vi "SV TDMS Write Waveform (SGL) (N Ch).vi"(0 "tdms file":refnum<k34>, 1 "write channel properties":bool=TRUE, 5 "group name in":string="Waveforms", 7 "channel names in":string[](array[string]), 9 "scaled signals":waveform(sgl)[](array[waveform]), 11 "error in":errorcluster) -> (4 "tdms file out":refnum<k34>, 6 "group name out":string, 8 "channel names out":string[](array[string]), 15 "error out":errorcluster)   [LabVIEW 2017]
doc: "Writes data to the specified .tdms file in a format specific to the polymorphic instance. Wire data to the <B>scaled signal [EU]</B> input to determine the polymorphic instance to use or manually select the instance."
uses:
  <vilib>/addons/_NISVFA/_Shared subVIs/Controls/LV Datatypes.ctl
  <vilib>/addons/_NISVFA/_Shared subVIs/Controls/NI Function Type.ctl
  <vilib>/addons/_NISVFA/_Shared subVIs/Controls/NI Function SubType.ctl
  <vilib>/addons/_NISVFA/_Shared subVIs/Controls/svc_X-Axis Units.ctl
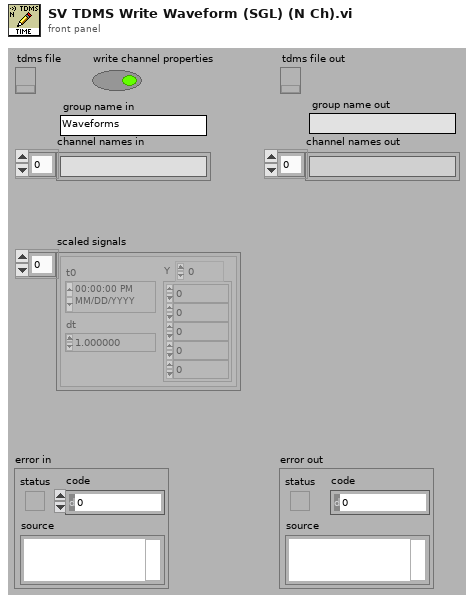
[diagram p1: front panel]
types:
  T1 = typedef "NI Function Type.ctl" = u16
  T2 = typedef "NI Function SubType.ctl" = u16
  T3 = typedef "svc_X-Axis Units.ctl" = u16
  T4 = cluster{"function type":T1, "function subtype":T2, "X-dimension":T3}
  T5 = cluster{"X-axis label":string, "X-unit string":string, "Y-axis label":string, "Y-unit string":string}
  T6 = typedef "LV Datatypes.ctl" = i32
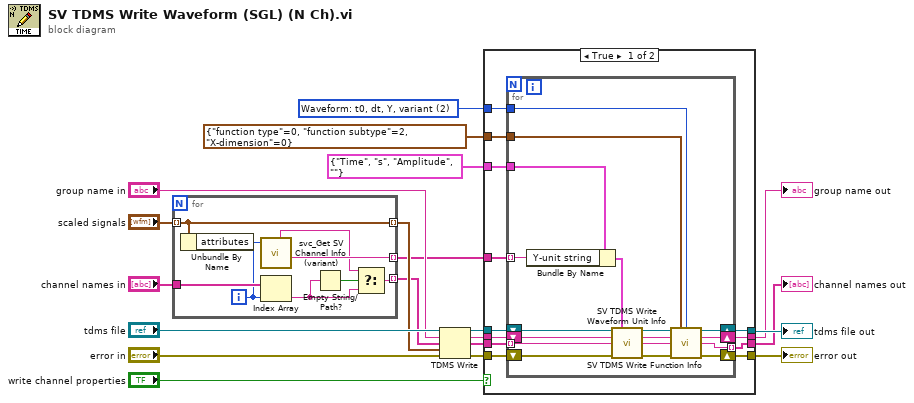
[diagram p0: block diagram]
diagram:
  w1 = T6 2 items=["String: abc"=-2, "Boolean: True or False"=-1, "Scalar: y"=0, "Array: Y"=1, "Waveform: t0, dt, Y, variant"=2, "Cluster: x0, dx, Y"=3, "Cluster: X, Y"=4, "Waterfall"=5, "Colormap"=6] ("LabVIEW datatype")
  n1 = for {
    tunnel: "scaled signals" -> [w22] mode=indexing
    tunnel: [w22] -> w7 mode=indexing
    tunnel: [w29] -> w6 mode=indexing
    tunnel: "channel names in" -> [w27]
    tunnel: [w25] -> w4 mode=indexing
    i -> [w26]
    n2 = Unbundle By Name(w22) -> ("attributes"=w21:variant)
    n3 = call <vilib>:"svc_Get SV Channel Info (variant).vi"("channel index"=w26, "attributes"=w21) -> ("unit label"=w29:string, "channel name"=w28:string)  [unwired: 4 in, 4 out]
    n4 = Index Array(array=w27, index=w26) -> (element=w23:string)
    n5 = Empty String/Path?(string/path=w23) -> (empty?=w24:bool)
    n6 = Select(t=w28, s=w24, f=w23) -> (s? t:f=w25:string)
  }
  n7 = TDMS Write(0:"tdms file", 5:"group name in", 7:w4, 9:w7, 11:"error in") -> (4:w15:refnum<k34>, 6:w13:string, 8:w12:string[], 15:w10:errorcluster)  [unwired: 1 in]
  n8 = case shown="True" "write channel properties" {
    tunnel: [w41 w62] -> w20
    tunnel: [w40 w61] -> w19
    tunnel: w10 -> [w39 w61]
    tunnel: w15 -> [w38 w62]
    tunnel: [w31 w60] -> w18
    tunnel: [w30 w59] -> w17
    tunnel: w13 -> [w37 w60]
    tunnel: w12 -> [w36 w59]
    tunnel: w6 -> [w35 _]
    tunnel: T4 {"function type"=0, "function subtype"=2, "X-dimension"=0} ("function info") -> [w34 _]
    tunnel: T5 {"X-axis label"="Time", "X-unit string"="s", "Y-axis label"="Amplitude", "Y-unit string"=""} ("unit info") -> [w33 _]
    tunnel: w1 -> [w32 _]
    frame True {
      n9 = for {
        shift-right: [w45] -> w41
        shift-left: w38 -> [w53]
        shift-right: [w42] -> w40
        shift-left: w39 -> [w50]
        tunnel: w36 -> [w51] mode=indexing
        tunnel: w35 -> [w56] mode=indexing
        tunnel: w34 -> [w58]
        tunnel: w33 -> [w57]
        tunnel: w32 -> [w54]
        tunnel: [w43] -> w30 mode=indexing
        shift-right: [w44] -> w31
        shift-left: w37 -> [w52]
        n10 = Bundle By Name(cluster=w57, "Y-unit string"=w56) -> (w55:T5)
        n11 = call <vilib>:"SV TDMS Write Waveform Unit Info.vi"("tdms file"=w53, "unit info"=w55, "group name"=w52, "channel name"=w51, "error in (no error)"=w50) -> ("tdms file out"=w49:refnum<k34>, "group name out"=w48:string, "channel name out"=w47:string, "error out"=w46:errorcluster)  [unwired: 7 in]
        n12 = call <vilib>:"SV TDMS Write Function Info.vi"("tdms file in"=w49, "function info"=w58, "LabVIEW datatype"=w54, "group name"=w48, "channel name"=w47, "error in (no error)"=w46) -> ("tdms file out"=w45:refnum<k34>, "group name out"=w44:string, "channel name out"=w43:string, "error out"=w42:errorcluster)  [unwired: 6 in]
      }
    }
    frame False {
    }
  }
  "tdms file out" <- w20
  "error out" <- w19
  "channel names out" <- w17
  "group name out" <- w18
